vi "Exit.vi"(7 "Exit Notifier":refnum<notifier>, 8 "error in":errorcluster, 10 "UI Queue":refnum<queue>, 11 "Message Queue":refnum<queue>) -> (0 "error out":errorcluster)   [LabVIEW 2014, in "DAQ.lvlib"]
uses:
  DAQ.lvlib
  support/Message Queue/Message Queue.lvlib
  support/Message Queue/Enqueue Message (Single).vi
  support/Message Queue/Message Cluster.ctl
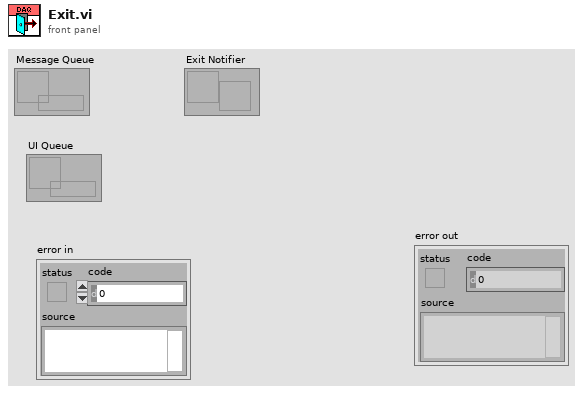
[diagram p1: front panel]
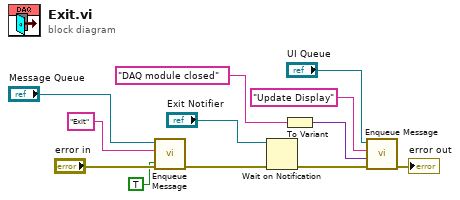
[diagram p0: block diagram]
diagram:
  n1 = call-poly "Enqueue Message.vi"("Priority Message? (F)"=TRUE, "error in (no error)"="error in", "Message"="Exit", "Message Queue"="Message Queue") -> ("error out"=w8:errorcluster)  [unwired: 6 in, 1 out]
  n2 = Wait on Notification(notifier="Exit Notifier", error in (no error)=w8) -> (error out=w6:errorcluster)  [unwired: 2 in, 3 out]
  n3 = To Variant(anything="DAQ module closed" ("Message")) -> (Variant=w2:variant)
  n4 = call-poly "Enqueue Message.vi"("error in (no error)"=w6, "Message Data"=w2, "Message"="Update Display", "Message Queue"="UI Queue") -> ("error out"=→"error out":errorcluster)  [unwired: 6 in, 1 out]
